vi "read.vi"(0 "MB_TCP session in":refnum<class "MB_Master_TCP.lvclass">, 3 "error in":errorcluster) -> (7 "MB_TCP session out":refnum<class "MB_Master_TCP.lvclass">, 10 "error out":errorcluster)   [LabVIEW 2025, in "TanksPlcDriver.lvlib"]
uses:
  TanksPlcDriver.lvlib
  <vilib>/platform/TimedLoop/XDataNode/XDataNode.xnode
  <vilib>/Platform/TimedLoop/XDataNode/nitl_modes.ctl
  <vilib>/Platform/TimedLoop/XDataNode/XDNodeRunTimeDep.lvlib
  <vilib>/Platform/TimedLoop/XDataNode/wakeup.ctl
  <vilib>/Platform/TimedLoop/XDataNode/timing_clust.ctl
  <vilib>/Plasmionique/MB Master/MB Master.lvlib
  <vilib>/Plasmionique/MB Master/MB_Master_TCP/MB_Master_TCP.lvclass
  TypeDefs/ReadData.ctl
panel:
  out "Read Data":T1 {"Conductivity [uS/cm]" format="%#_f"; "Pressure [bar]" format="%#_f"; "PH" format="%#_f"; "Water Level [l]" format="%#_f"; "Temperature [°C]" format="%#_f"}
  in  "IP Address":string="192.168.0.28"
  in  "Initialize":bool
  out "Response [ms]":dbl format="%.1f"
  in  "Period [ms]":i32=200 min=1 max=60000
  in  "Read Continuous":bool
  # "Driver Testing"
  # "Debug values...."
  # "Tanks  Driver V0.10\nRead"
  # "10.06.2025"
  # "Blaz Kelbl"
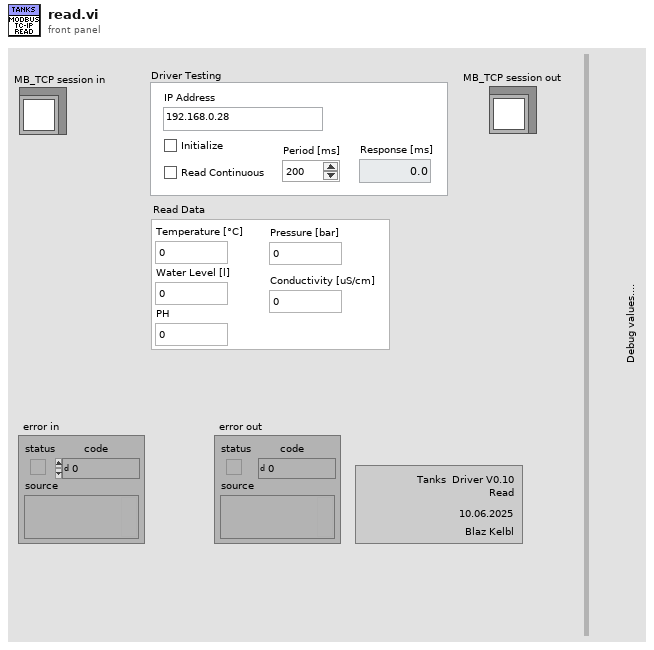
[diagram p1: front panel]
types:
  T1 = typedef "TanksPlcDriver.lvlib/ReadData.ctl" = cluster{"Temperature [°C]":dbl, "Water Level [l]":dbl, "PH":dbl, "Pressure [bar]":dbl, "Conductivity [uS/cm]":dbl}
  T2 = typedef "XDNodeRunTimeDep.lvlib/timing_clust.ctl" = cluster{"Expected End [f-1]":u64, "Actual End [f-1]":u64, "Finished Late? [f-1]":bool, "Expected End [i-1]":u64, "Actual End [i-1]":u64, "Finished Late? [i-1]":bool, "Expected Start [i]":u64, "Actual Start [i]":u64, "Expected Start [f]":u64, "Actual Start [f]":u64, "Source Name":string, "Structure Name":string, "Period":i64, "Deadline":i64, "Offset":i64, "Start":i64, "Priority":i32, "Timeout":i32, "Mode":T3, "Wakeup Reason":T4, "Error":errorcluster, "Source Type":string, "Secondary Source Type":string, "Global End Time":u64, "Global Start Time":u64, "Frame Duration":u64, "Iteration Duration":u64, "Assigned CPU":i32, "I/O Scan Engine Mode":u32}
  T3 = typedef "XDNodeRunTimeDep.lvlib/nitl_modes.ctl" = enum32{"No Change", "Process missed periods, maintain original phase", "Discard missed periods, maintain original phase", "Process missed periods, ignore original phase", "Discard missed periods, ignore original phase"}
  T4 = typedef "XDNodeRunTimeDep.lvlib/wakeup.ctl" = enum32{"Normal", "Aborted", "Asynchronous wakeup", "Timing source error", "Timed loop error", "Timeout"}
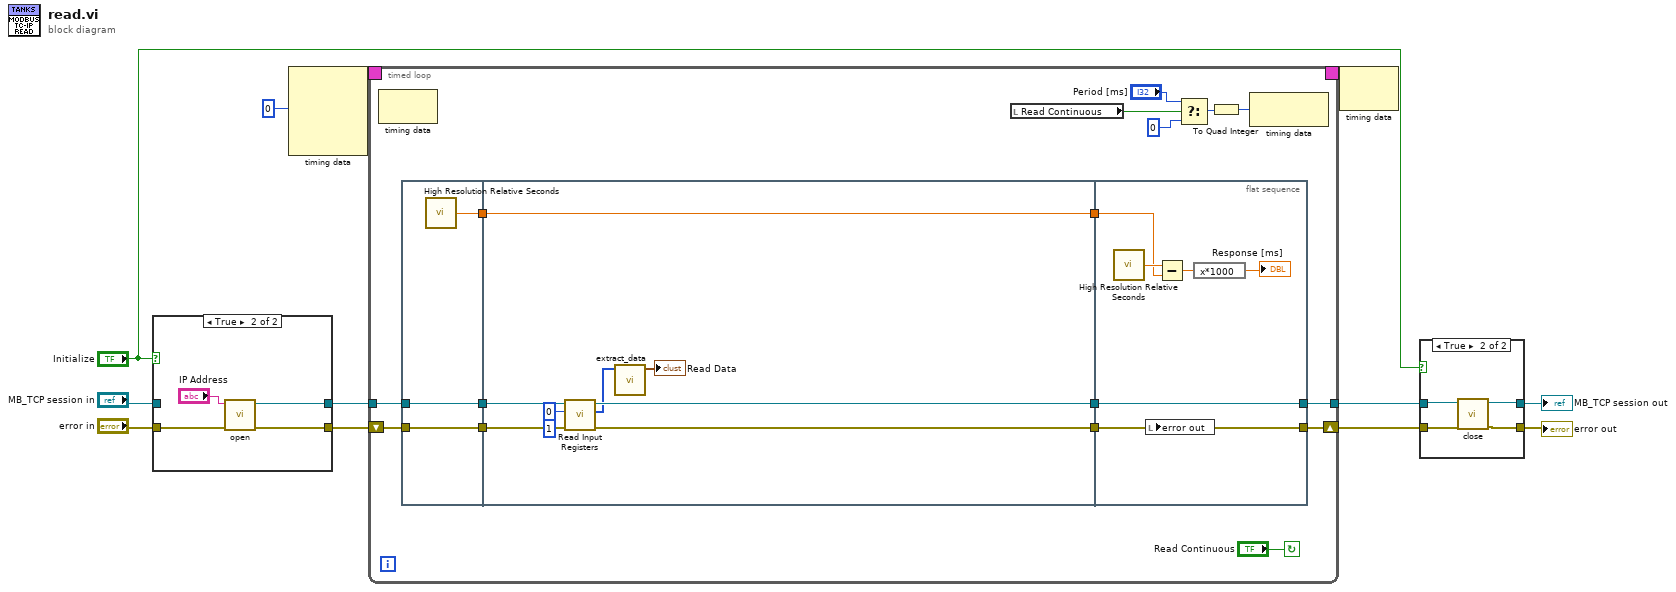
[diagram p0: block diagram]
diagram:
  n1 = case shown="True" "Initialize" {
    tunnel: "error in" -> [w13 w16]
    tunnel: [w13 w17] -> w7
    tunnel: [w14 w15] -> w6
    tunnel: "MB_TCP session in" -> [w14 _]
    frame False {
    }
    frame True {
      n2 = call "open.vi"("error in"=w16, "IP Address"="IP Address") -> ("error out"=w17:errorcluster, "MB_TCP session out"=w15:refnum<class "MB_Master_TCP.lvclass">)  [unwired: 8 in]
    }
  }
  n3 = node-c288(i64 0 ("Period")) -> (w12:T2)  [unwired: 3 in]
  n4 = timed-loop {
    timing: w12 -> [_]
    timing-out: [_] -> w11
    tunnel: w6 -> [w28]
    tunnel: [w27] -> w4
    shift-right: [w23] -> w3
    shift-left: w7 -> [w26]
    stop <- "Read Continuous" continue-if-true
    n5 = node-c288() -> ()  [unwired: 1 in, 1 out]
    n6 = flat-sequence {
      tunnel: w26 -> [w36]
      tunnel: w28 -> [w37]
      tunnel: [w37] -> w22
      tunnel: [w36] -> w21
      tunnel: [w35] -> w19
      tunnel: [w43] -> w25
      tunnel: [w45] -> w24
      tunnel: w22 -> [w42]
      tunnel: w21 -> [w44]
      tunnel: [w46] -> w20
      tunnel: w19 -> [w46]
      tunnel: [w51] -> w23
      tunnel: [w52] -> w27
      tunnel: w25 -> [w52]
      tunnel: w24 -> [w51]
      tunnel: w20 -> [w47]
      frame #0 {
        n7 = call <vilib>:"High Resolution Relative Seconds.vi"() -> ("relative seconds"=w35:dbl)
      }
      frame #1 {
        n8 = call <vilib>:"Read Input Registers.vi"("error in (no error)"=w44, "quantity"=u16 1, "starting address"=u16 0, "MB session in"=w42) -> ("error out"=w45:errorcluster, "Registers"=w41:u16[], "MB session out"=w43:refnum<class "MB_Master_TCP.lvclass">)  [unwired: 5 in]
        n9 = call "extract_data.vi"("Data IN"=w41) -> ("Read Data"=→"Read Data":T1)  [unwired: 10 in]
      }
      frame #2 {
        n10 = call <vilib>:"High Resolution Relative Seconds.vi"() -> ("relative seconds"=w50:dbl)
        n11 = local write "error out"(w51) -> ()
        n12 = Subtract(x=w50, y=w47) -> (x-y=w49:dbl)
        n13 = expression code="x*1000"(w49) -> (→"Response [ms]":dbl)
      }
    }
    n14 = local read "Read Continuous"() -> (w32:bool)
    n15 = Select(t="Period [ms]", s=w32, f=0) -> (s? t:f=w30:i32)
    n16 = To Quad Integer(1:w30) -> (0:w29:i64)
    n17 = node-c288(w29) -> ()  [unwired: 1 out]
  }
  n18 = node-c288(w11) -> ()  [unwired: 1 out]
  n19 = case shown="True" "Initialize" {
    tunnel: w4 -> [w58 w59]
    tunnel: w3 -> [w57 w61]
    tunnel: [w58 w59] -> w2
    tunnel: [w57 w60] -> w1
    frame False {
    }
    frame True {
      n20 = call "close.vi"("error in"=w61, "MB_TCP session in"=w59) -> ("error out"=w60:errorcluster)  [unwired: 9 in]
    }
  }
  "MB_TCP session out" <- w2
  "error out" <- w1
